vi "communicate gpib.vi"() -> ()   [LabVIEW 2014]
panel:
  in  "Send command 2":bool
  in  "GPIB command string":string
  out "finished moving?":bool
  in  "Send command":bool
  in  "stop":bool
  out "GPIB output string":string
  in  "GPIB querry string":string
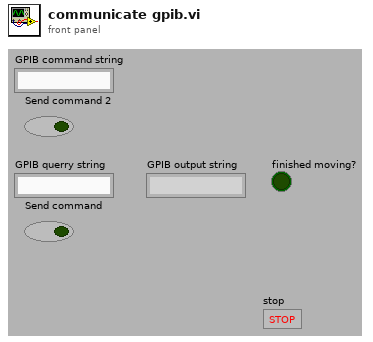
[diagram p1: front panel]
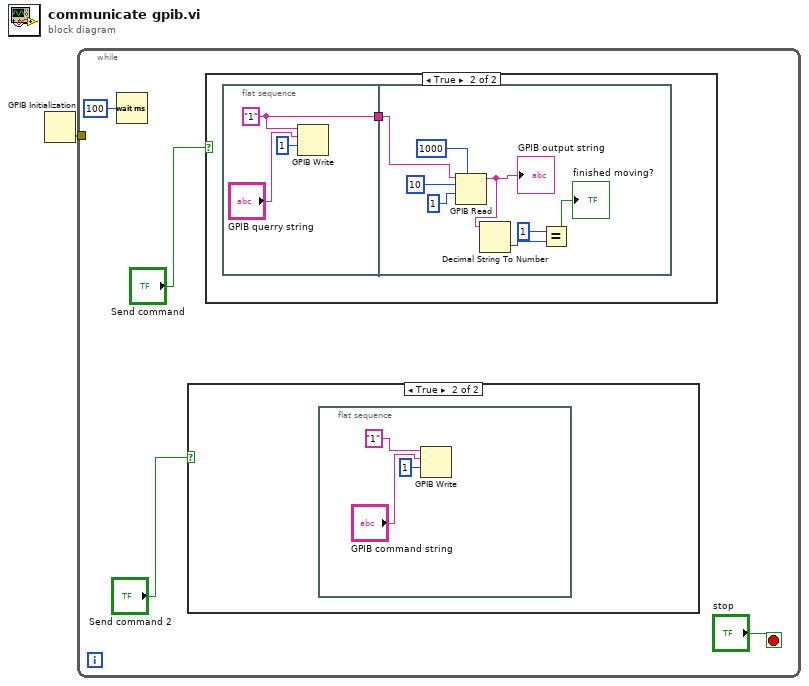
[diagram p0: block diagram]
diagram:
  n1 = GPIB Initialization() -> (0:w1:errorcluster)  [unwired: 7 in]
  n2 = while {
    tunnel: w1 -> [_]
    stop <- "stop" stop-if-true
    n3 = Wait (ms)(milliseconds to wait=u32 100) -> ()  [unwired: 1 out]
    n4 = case shown="True" "Send command 2" {
      frame False {
      }
      frame True {
        n5 = flat-sequence {
          frame #0 {
            n6 = GPIB Write(0:"1" ("address string"), 1:"GPIB command string", 2:i16 1 ("mode (0)")) -> ()  [unwired: 2 in, 2 out]
          }
        }
      }
    }
    n7 = case shown="True" "Send command" {
      frame False {
      }
      frame True {
        n8 = flat-sequence {
          tunnel: [w10] -> w9
          tunnel: w9 -> [w17]
          frame #0 {
            w10 = "1" ("address string")
            n9 = GPIB Write(0:w10, 1:"GPIB querry string", 2:i16 1 ("mode (0)")) -> ()  [unwired: 2 in, 2 out]
          }
          frame #1 {
            n10 = GPIB Read(0:w17, 1:10 ("byte count"), 2:i16 1 ("mode (0)"), 4:1000 ("timeout ms (488.2 global)")) -> (5:w16:string)  [unwired: 1 in, 2 out]
            "GPIB output string" <- w16
            n11 = Decimal String To Number(string=w16) -> (number=w15:i32)  [unwired: 2 in, 1 out]
            n12 = Equal?(x=1, y=w15) -> (x = y?=→"finished moving?":bool)
          }
        }
      }
    }
  }
